vi "SHsUmrechnen-15-07-17.vi"(6 "TemperaturenSH[V]":dbl[](array[numeric]), 7 "SpannungenSH[V]":dbl[](array[numeric]), 9 "Traps/MachKoeff2":dbl[](array[numeric]), 10 "Traps/MachKoeff1":dbl[](array[numeric]), 11 "Traps/MachKoeff0":dbl[](array[numeric])) -> (2 "SpannungenSH":T1 {"setpoint" format="%.23g"; "setpoint" format="%.23g"; "[2]" format="%.23g"; "[3]" format="%.23g"; "[4]" format="%.23g"; "[5]" format="%.23g"}, 3 "TemperaturenSH[°C]":dbl[](array[numeric]))   [LabVIEW 2010]
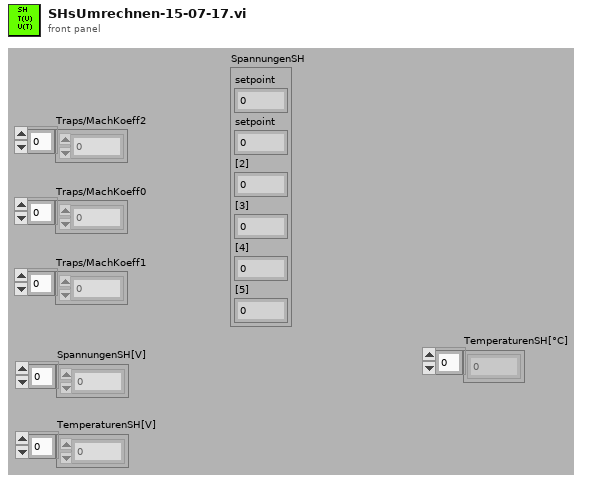
[diagram p1: front panel]
types:
  T1 = cluster{"setpoint":fxp<+/-,26,5>, "setpoint":fxp<+/-,26,5>, "[2]":fxp<+/-,26,5>, "[3]":fxp<+/-,26,5>, "[4]":fxp<+/-,26,5>, "[5]":fxp<+/-,26,5>}
  T2 = cluster{"[0]":fxp<+/-,26,5>, "[1]":fxp<+/-,26,5>, "[2]":fxp<+/-,26,5>, "[3]":fxp<+/-,26,5>, "[4]":fxp<+/-,26,5>, "[5]":fxp<+/-,26,5>}
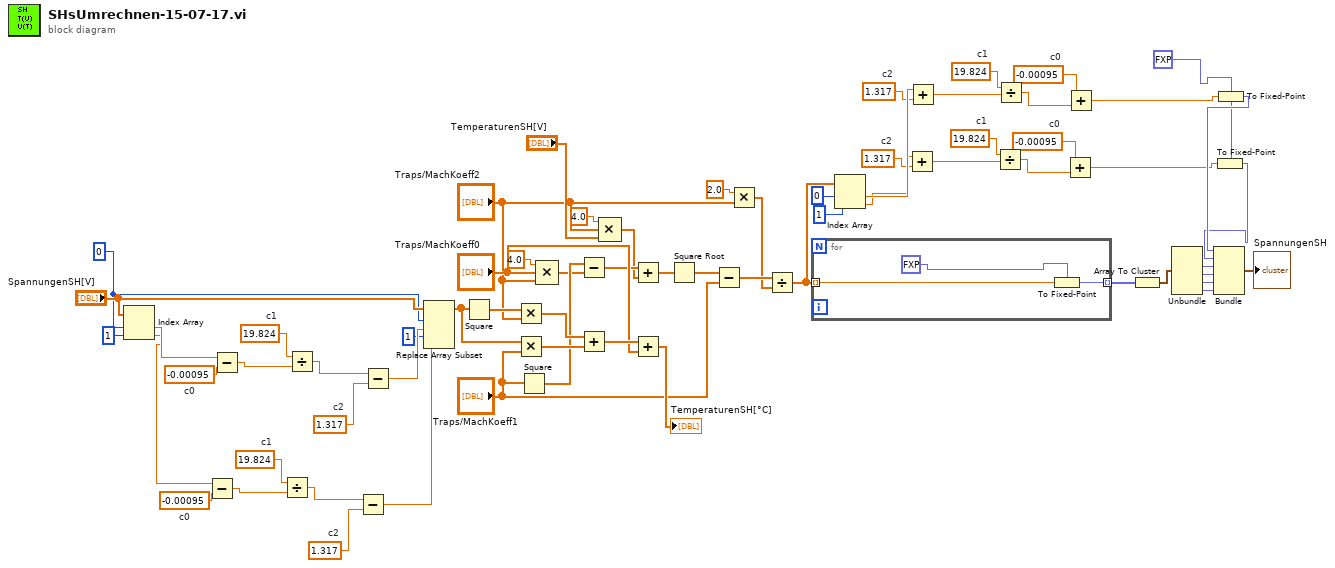
[diagram p0: block diagram]
diagram:
  w3 = fxp<+/-,26,5> 0.0 ("setpoint")
  w8 = -0.00095  # c0
  w10 = 19.824  # c1
  w11 = 1.317  # c2
  w15 = -0.00095  # c0
  w17 = 19.824  # c1
  w18 = 1.317  # c2
  w24 = 1.317  # c2
  w27 = 19.824  # c1
  w28 = -0.00095  # c0
  w31 = 1.317  # c2
  w34 = 19.824  # c1
  w35 = -0.00095  # c0
  w38 = 0 ("index")
  n1 = Index Array(array="SpannungenSH[V]", index #1=w38, index #2=1 ("index")) -> (element #1=w36:dbl, element #2=w22:dbl)
  n2 = Subtract(x=w22, y=w28) -> (x-y=w26:dbl)
  n3 = Subtract(x=w36, y=w35) -> (x-y=w33:dbl)
  n4 = Divide(x=w27, y=w26) -> (x/y=w25:dbl)
  n5 = Divide(x=w34, y=w33) -> (x/y=w32:dbl)
  n6 = Subtract(x=w25, y=w24) -> (x-y=w21:dbl)
  n7 = Subtract(x=w32, y=w31) -> (x-y=w30:dbl)
  n8 = Replace Array Subset(array="SpannungenSH[V]", new element #1=w30, index #1=w38, new element #2=w21, index #2=1 ("index")) -> (w37:dbl[])
  n9 = Square(x=w37) -> (x^2=w63:dbl[])
  n10 = Multiply(x=w63, y="Traps/MachKoeff2") -> (x*y=w64:dbl[])
  n11 = Multiply(x=w37, y="Traps/MachKoeff1") -> (x*y=w65:dbl[])
  n12 = Square(x="Traps/MachKoeff1") -> (x^2=w57:dbl[])
  n13 = Compound Arithmetic op=MULTIPLY(4.0, "Traps/MachKoeff0", "Traps/MachKoeff2") -> (w56:dbl[])
  n14 = Subtract(x=w57, y=w56) -> (x-y=w55:dbl[])
  n15 = Add(x=w64, y=w65) -> (x+y=w66:dbl[])
  n16 = Compound Arithmetic op=MULTIPLY(4.0, "Traps/MachKoeff2", "TemperaturenSH[V]") -> (w54:dbl[])
  n17 = Add(x=w55, y=w54) -> (x+y=w53:dbl[])
  n18 = Add(x=w66, y="Traps/MachKoeff0") -> (x+y=→"TemperaturenSH[°C]":dbl[])
  n19 = Square Root(x=w53) -> (sqrt(x)=w1:dbl[])
  n20 = Subtract(x=w1, y="Traps/MachKoeff1") -> (x-y=w51:dbl[])
  n21 = Multiply(x=2.0, y="Traps/MachKoeff2") -> (x*y=w48:dbl[])
  n22 = Divide(x=w51, y=w48) -> (x/y=w46:dbl[])
  n23 = for {
    tunnel: w46 -> [w69] mode=indexing
    tunnel: [w68] -> w45 mode=indexing
    n24 = To Fixed-Point(fixed-point type=fxp<+/-,26,5> 0.0 ("setpoint"), number=w69) -> (fixed-point=w68:fxp<+/-,26,5>)
  }
  n25 = Index Array(array=w46, index #1=0 ("index"), index #2=1 ("index")) -> (element #1=w19:dbl, element #2=w5:dbl)
  n26 = Add(x=w5, y=w11) -> (x+y=w9:dbl)
  n27 = Add(x=w19, y=w18) -> (x+y=w16:dbl)
  n28 = Divide(x=w10, y=w9) -> (x/y=w7:dbl)
  n29 = Divide(x=w17, y=w16) -> (x/y=w14:dbl)
  n30 = Add(x=w8, y=w7) -> (x+y=w6:dbl)
  n31 = Add(x=w15, y=w14) -> (x+y=w13:dbl)
  n32 = Array To Cluster(array=w45) -> (cluster=w44:T2)
  n33 = Unbundle(w44) -> ("[2]"=w43:fxp<+/-,26,5>, "[3]"=w42:fxp<+/-,26,5>, "[4]"=w41:fxp<+/-,26,5>, "[5]"=w40:fxp<+/-,26,5>)  [unwired: 2 out]
  n34 = To Fixed-Point(fixed-point type=w3, number=w6) -> (fixed-point=w4:fxp<+/-,26,5>)
  n35 = To Fixed-Point(fixed-point type=w3, number=w13) -> (fixed-point=w12:fxp<+/-,26,5>)
  n36 = Bundle("setpoint"=w12, "setpoint"=w4, "[2]"=w43, "[3]"=w42, "[4]"=w41, "[5]"=w40) -> (→"SpannungenSH":T1)  [unwired: 1 in]
